vi "circular buffer.vi"(0 "StreamToWrite":u8[](array[numeric]), 7 "NumberOfBytes":i32, 11 "ByteToWrite":u8, 13 "Enum":T1(ring)) -> (4 "OutputBytes":u8[](array[numeric]), 8 "Output":i32)   [LabVIEW 2010]
panel:
  out "Buffer":u8[](array[numeric])
  out "Tail":i32
  out "Head":i32
  # "Points ot the next available position"
  # "Points to the last occupied position"
  # "Note: If they are equal, no data are available"
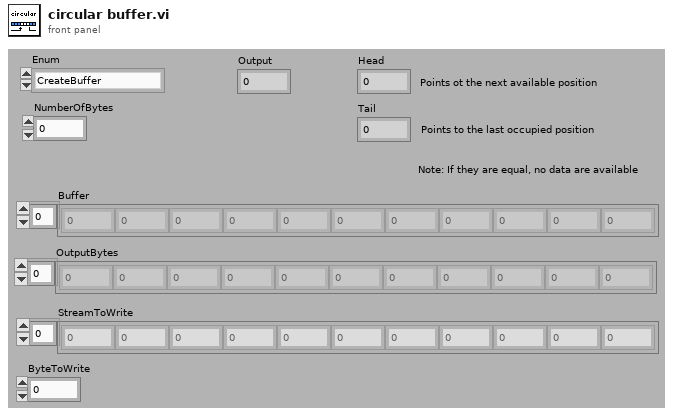
[diagram p1: front panel]
types:
  T1 = enum16{"CreateBuffer", "WriteBytes", "WriteByte", "AvailableMemory", "OccupiedMemory", "CheckBytes", "ReadBytes"}
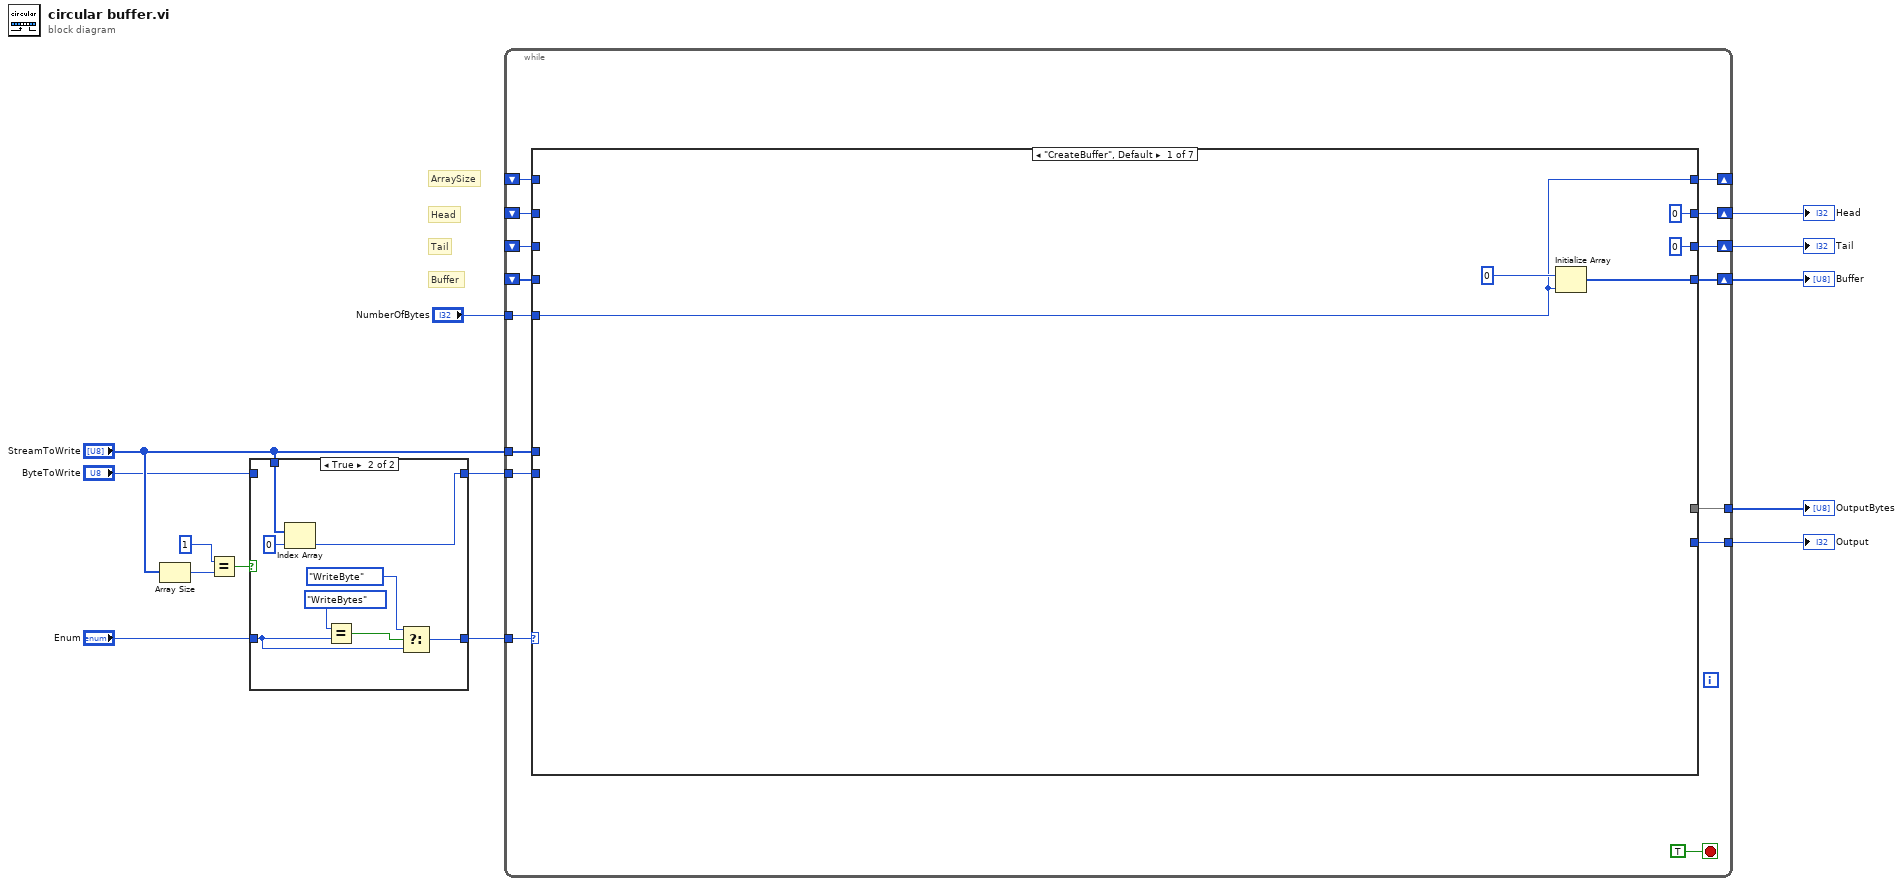
[diagram p0: block diagram]
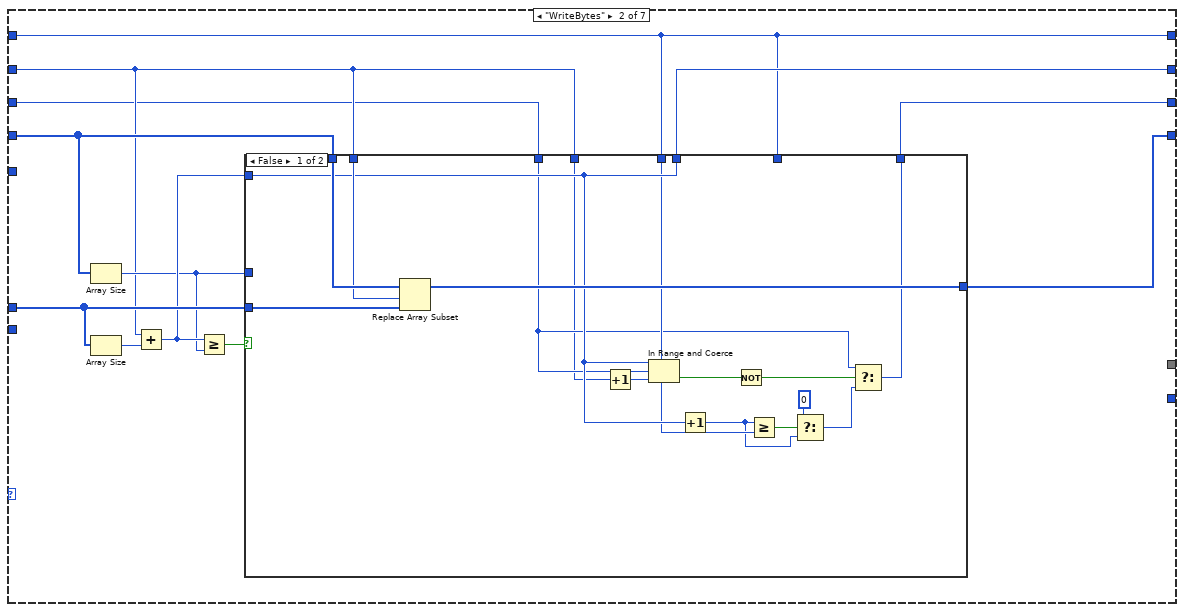
[diagram p3: hidden frame]
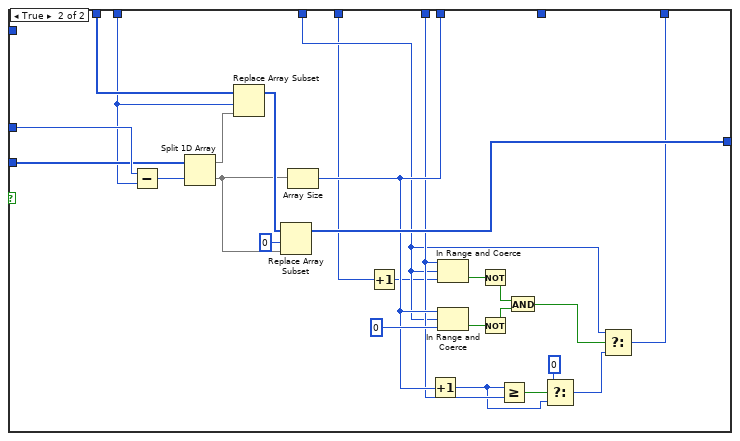
[diagram p4: hidden frame]
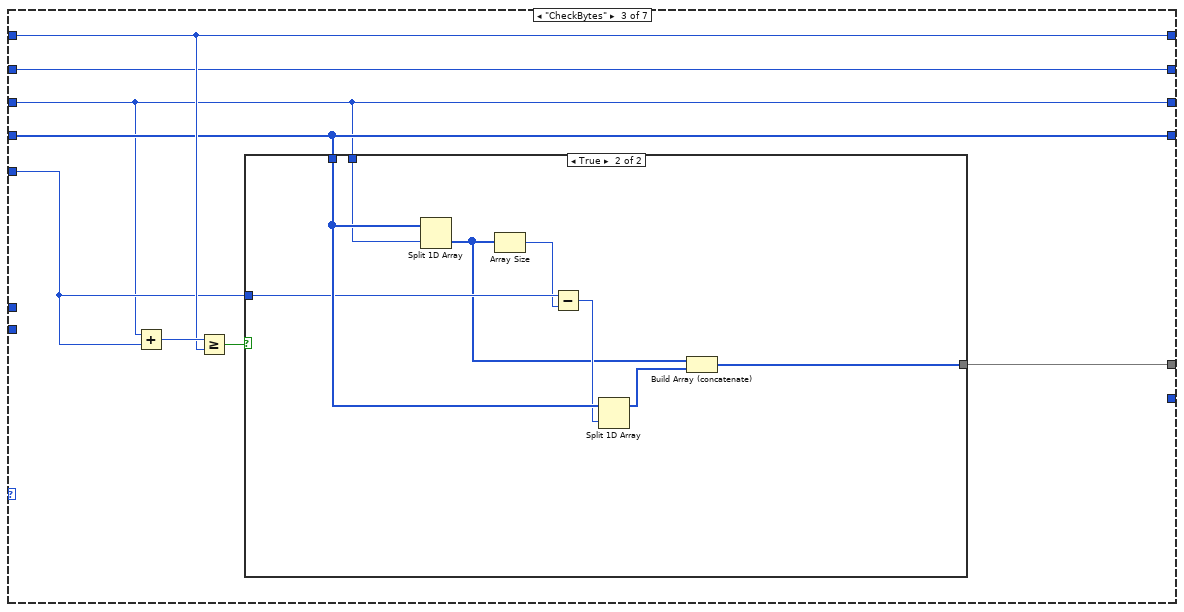
[diagram p5: hidden frame]
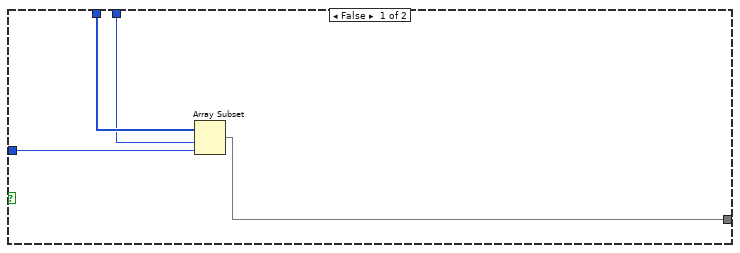
[diagram p6: hidden frame]
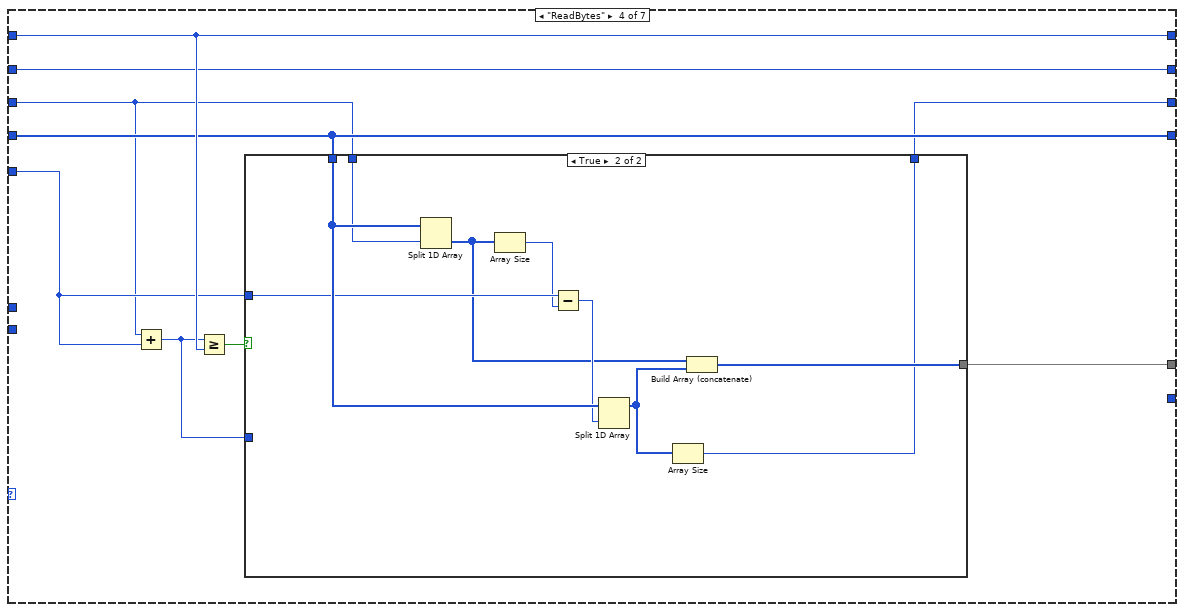
[diagram p7: hidden frame]
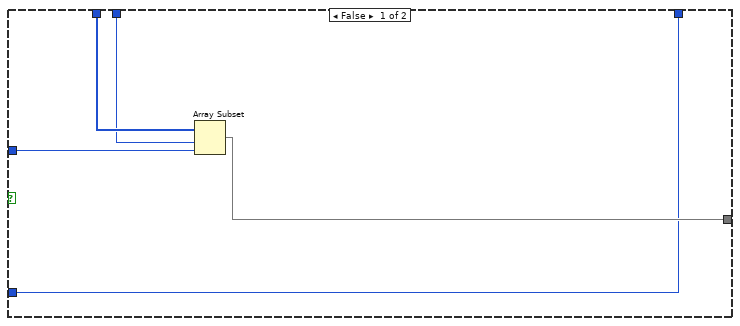
[diagram p8: hidden frame]
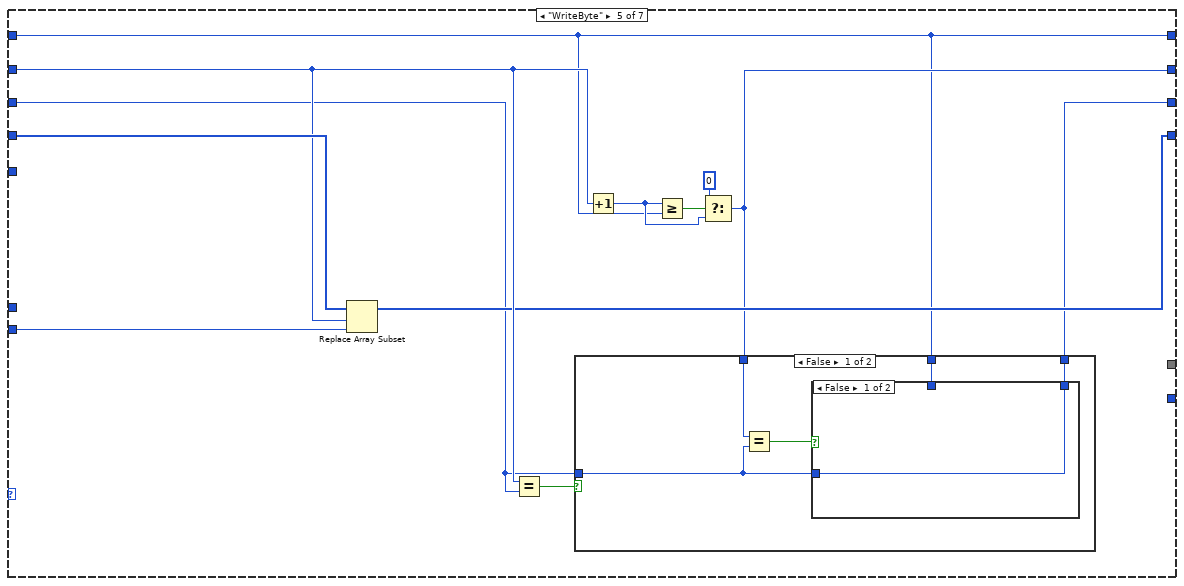
[diagram p9: hidden frame]
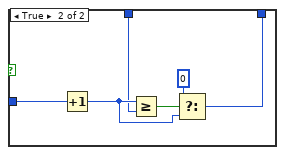
[diagram p10: hidden frame]
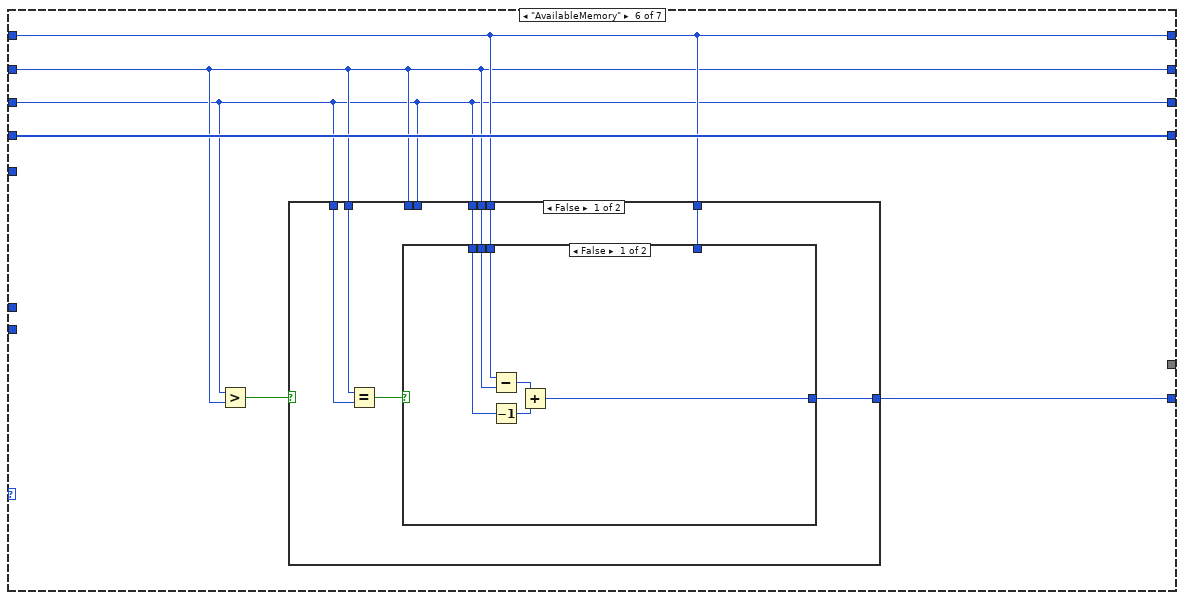
[diagram p12: hidden frame]
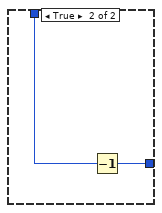
[diagram p13: hidden frame]
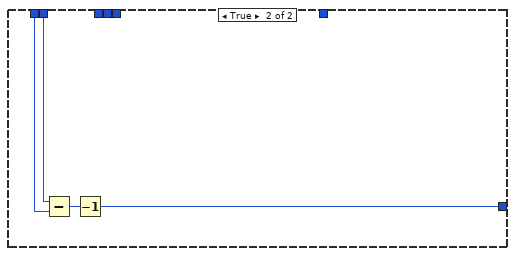
[diagram p14: hidden frame]
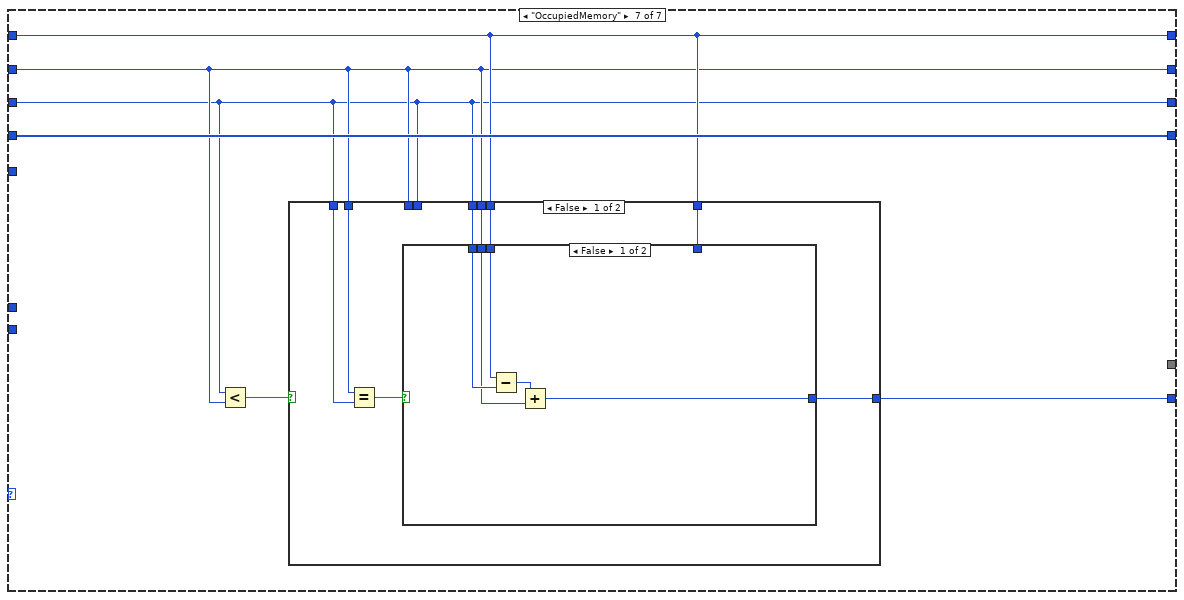
[diagram p15: hidden frame]
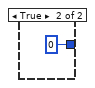
[diagram p16: hidden frame]
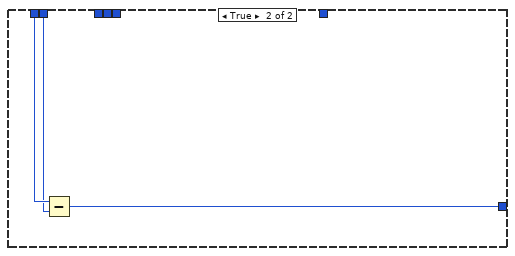
[diagram p17: hidden frame]
diagram:
  # "Buffer"
  # "Tail"
  # "Head"
  # "ArraySize"
  n1 = Array Size(array="StreamToWrite") -> (size(s)=w11:i32)
  n2 = Equal?(x=1, y=w11) -> (x = y?=w8:bool)
  n3 = case shown="True" w8 {
    tunnel: "StreamToWrite" -> [_ w24]
    tunnel: [w16 w22] -> w7
    tunnel: "Enum" -> [w16 w20]
    tunnel: [w15 w19] -> w5
    tunnel: "ByteToWrite" -> [w15 _]
    frame False {
    }
    frame True {
      n4 = Index Array(array=w24, index=0) -> (element=w19:u8)
      n5 = Equal?(x=T1."WriteBytes", y=w20) -> (x = y?=w21:bool)
      n6 = Select(t=T1."WriteByte" ("x"), s=w21, f=w20) -> (s? t:f=w22:T1)
    }
  }
  n7 = while {
    shift-right: [w38] -> w14
    shift-left: _ -> [w39]
    tunnel: w7 -> [w37]
    shift-right: [w36] -> w13
    shift-left: _ -> [w34]
    shift-right: [w35] -> w12
    shift-left: _ -> [w33]
    shift-right: [w30] -> _
    shift-left: _ -> [w31]
    tunnel: "StreamToWrite" -> [w29]
    tunnel: w5 -> [w28]
    tunnel: [w27] -> w3
    tunnel: "NumberOfBytes" -> [w26]
    tunnel: [w25] -> w1
    stop <- TRUE stop-if-true
    n8 = case shown="\"CreateBuffer\", Default" w37 {
      tunnel: w39 -> [_ w54 w102 w124 w153 w172 w198]
      tunnel: [w44 w56 w102 w124 w147 w172 w198] -> w38
      tunnel: [0 ("Head") w49 w103 w125 w145 w168 w194] -> w36
      tunnel: [0 ("Tail") w48 w99 w119 w143 w167 w193] -> w35
      tunnel: w34 -> [_ w47 w103 w125 w148 w168 w194]
      tunnel: w33 -> [_ w46 w99 w120 w144 w167 w193]
      tunnel: w31 -> [_ w45 w104 w126 w142 w169 w195]
      tunnel: [w40 w45 w104 w126 w142 w169 w195] -> w30
      tunnel: w29 -> [_ w53 _ _ _ _ _]
      tunnel: w28 -> [_ _ _ _ w152 _ _]
      tunnel: [_ _ _ _ _ w170 w196] -> w27
      tunnel: w26 -> [w40 _ w101 w123 _ _ _]
      tunnel: [_ _ w100 w122 _ _ _] -> w25
      frame "CreateBuffer", Default {
        n9 = Initialize Array(u8 0, w40) -> (w44:u8[])
      }
      frame "WriteBytes" {
        n10 = Array Size(array=w54) -> (size(s)=w50:i32)
        n11 = Array Size(array=w53) -> (size(s)=w55:i32)
        n12 = Add(x=w47, y=w55) -> (x+y=w52:i32)
        n13 = Greater Or Equal?(x=w52, y=w50) -> (x >= y?=w51:bool)
        n14 = case shown="False" w51 {
          tunnel: [w72 w90] -> w56
          tunnel: w54 -> [w71 w95]
          tunnel: w47 -> [w70 w94]
          tunnel: w53 -> [w69 w97]
          tunnel: [w66 w79] -> w49
          tunnel: w52 -> [w66 _]
          tunnel: w50 -> [_ w98]
          tunnel: w45 -> [_ _]
          tunnel: [w67 w77] -> w48
          tunnel: w47 -> [w58 w74]
          tunnel: w46 -> [w59 w76]
          tunnel: w45 -> [w65 w78]
          frame False {
            n15 = Replace Array Subset "Replace Array Subset"(array=w71, new element=w69, index=w70) -> (w72:u8[])
            n16 = Increment(x=w58) -> (x+1=w57:i32)
            n17 = In Range and Coerce(upper limit=w66, x=w59, lower limit=w57) -> (In Range?=w68:bool)  [unwired: 1 out]
            n18 = Increment(x=w66) -> (x+1=w63:i32)
            n19 = Not(x=w68) -> (.not. x?=w60:bool)
            n20 = Greater Or Equal?(x=w63, y=w65) -> (x >= y?=w64:bool)
            n21 = Select(t=0, s=w64, f=w63) -> (s? t:f=w61:i32)
            n22 = Select(t=w59, s=w60, f=w61) -> (s? t:f=w67:i32)
          }
          frame True {
            n23 = Subtract(x=w98, y=w94) -> (x-y=w96:i32)
            n24 = Split 1D Array(array=w97, index=w96) -> (first subarray=w93:u8[], second subarray=w89:u8[])
            n25 = Replace Array Subset "Replace Array Subset"(array=w95, new element=w93, index=w94) -> (w92:u8[])
            n26 = Replace Array Subset "Replace Array Subset"(array=w92, new element=w89, index=0) -> (w90:u8[])
            n27 = Array Size(array=w89) -> (size(s)=w79:i32)
            n28 = Increment(x=w74) -> (x+1=w73:i32)
            n29 = Increment(x=w79) -> (x+1=w75:i32)
            n30 = In Range and Coerce(upper limit=w78, x=w76, lower limit=w73) -> (In Range?=w87:bool)  [unwired: 1 out]
            n31 = In Range and Coerce(upper limit=w79, x=w76, lower limit=0) -> (In Range?=w86:bool)  [unwired: 1 out]
            n32 = Not(x=w87) -> (.not. x?=w81:bool)
            n33 = Not(x=w86) -> (.not. x?=w82:bool)
            n34 = Greater Or Equal?(x=w75, y=w78) -> (x >= y?=w85:bool)
            n35 = And(x=w81, y=w82) -> (x .and. y?=w80:bool)
            n36 = Select(t=0, s=w85, f=w75) -> (s? t:f=w83:i32)
            n37 = Select(t=w76, s=w80, f=w83) -> (s? t:f=w77:i32)
          }
        }
      }
      frame "CheckBytes" {
        n38 = Add(x=w99, y=w101) -> (x+y=w106:i32)
        n39 = Greater Or Equal?(x=w106, y=w104) -> (x >= y?=w105:bool)
        n40 = case shown="True" w105 {
          tunnel: w102 -> [w110 w118]
          tunnel: w99 -> [w107 w114]
          tunnel: w101 -> [w109 w117]
          tunnel: [w108 w111] -> w100
          frame False {
            n41 = Array Subset(array=w110, index=w107, length=w109) -> (w108:u8[])
          }
          frame True {
            n42 = Split 1D Array(array=w118, index=w114) -> (second subarray=w113:u8[])  [unwired: 1 out]
            n43 = Array Size(array=w113) -> (size(s)=w115:i32)
            n44 = Subtract(x=w117, y=w115) -> (x-y=w116:i32)
            n45 = Split 1D Array(array=w118, index=w116) -> (first subarray=w112:u8[])  [unwired: 1 out]
            n46 = Build Array (concatenate)(w113, w112) -> (w111:u8[])
          }
        }
      }
      frame "ReadBytes" {
        n47 = Add(x=w120, y=w123) -> (x+y=w121:i32)
        n48 = Greater Or Equal?(x=w121, y=w126) -> (x >= y?=w127:bool)
        n49 = case shown="True" w127 {
          tunnel: w124 -> [w132 w141]
          tunnel: w120 -> [w129 w137]
          tunnel: w123 -> [w131 w140]
          tunnel: [w130 w135] -> w122
          tunnel: w121 -> [w128 _]
          tunnel: [w128 w133] -> w119
          frame False {
            n50 = Array Subset(array=w132, index=w129, length=w131) -> (w130:u8[])
          }
          frame True {
            n51 = Split 1D Array(array=w141, index=w137) -> (second subarray=w136:u8[])  [unwired: 1 out]
            n52 = Array Size(array=w136) -> (size(s)=w138:i32)
            n53 = Subtract(x=w140, y=w138) -> (x-y=w139:i32)
            n54 = Split 1D Array(array=w141, index=w139) -> (first subarray=w134:u8[])  [unwired: 1 out]
            n55 = Array Size(array=w134) -> (size(s)=w133:i32)
            n56 = Build Array (concatenate)(w136, w134) -> (w135:u8[])
          }
        }
      }
      frame "WriteByte" {
        n57 = Replace Array Subset "Replace Array Subset"(array=w153, new element=w152, index=w148) -> (w147:u8[])
        n58 = Equal?(x=w148, y=w144) -> (x = y?=w146:bool)
        n59 = Increment(x=w148) -> (x+1=w150:i32)
        n60 = Greater Or Equal?(x=w150, y=w142) -> (x >= y?=w151:bool)
        n61 = Select(t=0, s=w151, f=w150) -> (s? t:f=w145:i32)
        n62 = case shown="False" w146 {
          tunnel: w145 -> [w158 _]
          tunnel: w144 -> [w156 w166]
          tunnel: [w154 w166] -> w143
          tunnel: w142 -> [w155 _]
          frame False {
            n63 = Equal?(x=w158, y=w156) -> (x = y?=w157:bool)
            n64 = case shown="False" w157 {
              tunnel: w156 -> [w159 w162]
              tunnel: w155 -> [_ w161]
              tunnel: [w159 w160] -> w154
              frame False {
              }
              frame True {
                n65 = Increment(x=w162) -> (x+1=w164:i32)
                n66 = Greater Or Equal?(x=w164, y=w161) -> (x >= y?=w163:bool)
                n67 = Select(t=0, s=w163, f=w164) -> (s? t:f=w160:i32)
              }
            }
          }
          frame True {
          }
        }
      }
      frame "AvailableMemory" {
        n68 = Greater?(x=w167, y=w168) -> (0:w171:bool)
        n69 = case shown="False" w171 {
          tunnel: w167 -> [_ w192]
          tunnel: w168 -> [_ w191]
          tunnel: [w176 w189] -> w170
          tunnel: w168 -> [w180 _]
          tunnel: w167 -> [w179 _]
          tunnel: w169 -> [w177 _]
          tunnel: w169 -> [w175 _]
          tunnel: w168 -> [w174 _]
          tunnel: w167 -> [w173 _]
          frame False {
            n70 = Equal?(x=w180, y=w179) -> (x = y?=w178:bool)
            n71 = case shown="False" w178 {
              tunnel: w177 -> [_ w188]
              tunnel: [w181 w187] -> w176
              tunnel: w175 -> [w186 _]
              tunnel: w174 -> [w185 _]
              tunnel: w173 -> [w184 _]
              frame False {
                n72 = Subtract(x=w186, y=w185) -> (x-y=w183:i32)
                n73 = Decrement(x=w184) -> (x-1=w182:i32)
                n74 = Add(x=w183, y=w182) -> (x+y=w181:i32)
              }
              frame True {
                n75 = Decrement(x=w188) -> (x-1=w187:i32)
              }
            }
          }
          frame True {
            n76 = Subtract(x=w192, y=w191) -> (x-y=w190:i32)
            n77 = Decrement(x=w190) -> (x-1=w189:i32)
          }
        }
      }
      frame "OccupiedMemory" {
        n78 = Less?(x=w193, y=w194) -> (x < y?=w197:bool)
        n79 = case shown="False" w197 {
          tunnel: w193 -> [_ w214]
          tunnel: w194 -> [_ w215]
          tunnel: [w202 w213] -> w196
          tunnel: w194 -> [w206 _]
          tunnel: w193 -> [w205 _]
          tunnel: w195 -> [w203 _]
          tunnel: w195 -> [w201 _]
          tunnel: w194 -> [w200 _]
          tunnel: w193 -> [w199 _]
          frame False {
            n80 = Equal?(x=w206, y=w205) -> (x = y?=w204:bool)
            n81 = case shown="False" w204 {
              tunnel: w203 -> [_ _]
              tunnel: [w210 0] -> w202
              tunnel: w201 -> [w209 _]
              tunnel: w200 -> [w207 _]
              tunnel: w199 -> [w208 _]
              frame False {
                n82 = Subtract(x=w209, y=w208) -> (x-y=w211:i32)
                n83 = Add(x=w211, y=w207) -> (x+y=w210:i32)
              }
              frame True {
              }
            }
          }
          frame True {
            n84 = Subtract(x=w215, y=w214) -> (x-y=w213:i32)
          }
        }
      }
    }
  }
  "Head" <- w13
  "Tail" <- w12
  "Buffer" <- w14
  "Output" <- w3
  "OutputBytes" <- w1
